vi "DLS Profile.vi"(0 "GEA2 Reference In":refnum<k24>, 1 "Shift To":enum16{"Spin", "Agitate"}(ring), 2 "Input Bit":T3, 5 "GEA Inputs":T4={"Source"=228, "Destination"=192} {"Destination" format="%.0x"; "Source" format="%.0x"}, 7 "Standalone?":bool, 11 "Error In":errorcluster, 12 "Action":enum16{"Lock", "Unlock"}(ring), 13 "Co-efficient Data":T2) -> (4 "GEA2 Reference Out":refnum<k24>, 6 "Calc_Dry Load Size":dbl, 8 "Expected_Dry Load Size":dbl, 10 "Report Text":string, 14 "Pass/Fail":bool, 15 "Error Out":errorcluster)   [LabVIEW 2016, in "TLMB.lvlib"]
uses:
  Projects/TLMB.lvlib
  Q:/Common/DLLs/GEA3/GeaCommunication.dll
  Common/DLLs/GEA3/GeaCommunication.dll
  Common/LabVIEW GEA2 Toolkit/LabVIEW_GEA2_Toolkit.lvlibp/type defs/Source_Destination.ctl
  Control/DLS ERD Data.ctl
  TLMB Common/type defs/Drive Cycle Engine Request State.ctl
  Common/LabVIEW GEA2 Toolkit/LabVIEW_GEA2_Toolkit.lvlibp/type defs/ERD Read Data In.ctl
  Common/LabVIEW GEA2 Toolkit/LabVIEW_GEA2_Toolkit.lvlibp/type defs/Data Type.ctl
  Common/LabVIEW GEA2 Toolkit/LabVIEW_GEA2_Toolkit.lvlibp
panel:
  out "R1_DLS ERD Data":T1
  out "R1_Result Q5 Tranformation":dbl
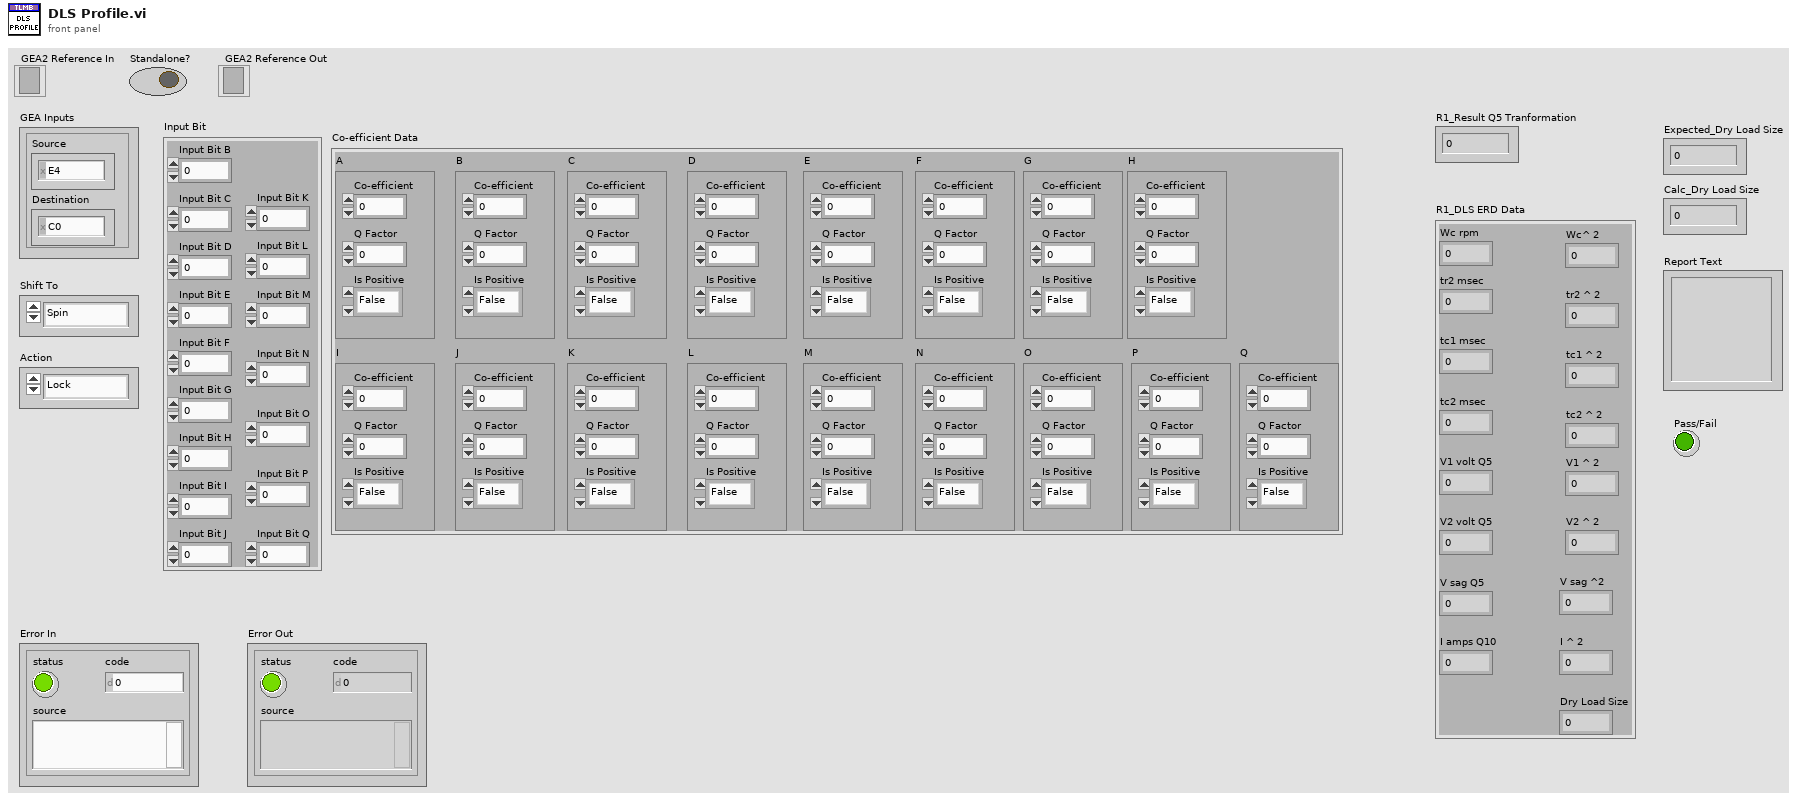
[diagram p1: front panel]
types:
  T1 = typedef "TLMB.lvlib/DLS ERD Data.ctl" = cluster{"Wc rpm":dbl, "tr2 msec":dbl, "tc1 msec":dbl, "tc2 msec":dbl, "V1 volt Q5":dbl, "V2 volt Q5":dbl, "I amps Q10":dbl, "Wc^ 2":dbl, "tr2 ^ 2":dbl, "tc1 ^ 2":dbl, "tc2 ^ 2":dbl, "V1 ^ 2":dbl, "V2 ^ 2":dbl, "I ^ 2":dbl, "V sag Q5":dbl, "V sag ^2":dbl, "Dry Load Size":dbl}
  T2 = cluster{"A":cluster{"Co-efficient":dbl, "Q Factor":dbl, "Is Positive":enum16{"False", "True"}}, "B":cluster{"Co-efficient":dbl, "Q Factor":dbl, "Is Positive":enum16{"False", "True"}}, "C":cluster{"Co-efficient":dbl, "Q Factor":dbl, "Is Positive":enum16{"False", "True"}}, "D":cluster{"Co-efficient":dbl, "Q Factor":dbl, "Is Positive":enum16{"False", "True"}}, "E":cluster{"Co-efficient":dbl, "Q Factor":dbl, "Is Positive":enum16{"False", "True"}}, "F":cluster{"Co-efficient":dbl, "Q Factor":dbl, "Is Positive":enum16{"False", "True"}}, "G":cluster{"Co-efficient":dbl, "Q Factor":dbl, "Is Positive":enum16{"False", "True"}}, "H":cluster{"Co-efficient":dbl, "Q Factor":dbl, "Is Positive":enum16{"False", "True"}}, "I":cluster{"Co-efficient":dbl, "Q Factor":dbl, "Is Positive":enum16{"False", "True"}}, "J":cluster{"Co-efficient":dbl, "Q Factor":dbl, "Is Positive":enum16{"False", "True"}}, "K":cluster{"Co-efficient":dbl, "Q Factor":dbl, "Is Positive":enum16{"False", "True"}}, "L":cluster{"Co-efficient":dbl, "Q Factor":dbl, "Is Positive":enum16{"False", "True"}}, "M":cluster{"Co-efficient":dbl, "Q Factor":dbl, "Is Positive":enum16{"False", "True"}}, "N":cluster{"Co-efficient":dbl, "Q Factor":dbl, "Is Positive":enum16{"False", "True"}}, "O":cluster{"Co-efficient":dbl, "Q Factor":dbl, "Is Positive":enum16{"False", "True"}}, "P":cluster{"Co-efficient":dbl, "Q Factor":dbl, "Is Positive":enum16{"False", "True"}}, "Q":cluster{"Co-efficient":dbl, "Q Factor":dbl, "Is Positive":enum16{"False", "True"}}}
  T3 = cluster{"Input Bit B":dbl, "Input Bit C":dbl, "Input Bit D":dbl, "Input Bit E":dbl, "Input Bit F":dbl, "Input Bit G":dbl, "Input Bit H":dbl, "Input Bit I":dbl, "Input Bit J":dbl, "Input Bit K":dbl, "Input Bit L":dbl, "Input Bit M":dbl, "Input Bit N":dbl, "Input Bit O":dbl, "Input Bit P":dbl, "Input Bit Q":dbl}
  T4 = typedef "LabVIEW_GEA2_Toolkit.lvlibp/Source_Destination.ctl" = cluster{"Source":u8, "Destination":u8}
  T5 = enum16{"EQ (==)", "NE (!=)", "GT (>)", "LT (<)", "GE (>=)", "LE (<=)", "GTLT(> <)", "GELE (>= <=)", "GELT (>= <)", "GTLE (> <=)", "LTGT (< >)", "LEGE (<= >=)", "LEGT (<= >)", "LTGE (< >=)", "No Comparison"}
  T6 = typedef "LabVIEW_GEA2_Toolkit.lvlibp/ERD Read Data In.ctl" = cluster{"ERD Number":u16, "Data Type":T7}
  T7 = typedef "LabVIEW_GEA2_Toolkit.lvlibp/Data Type.ctl" = enum16{"string", "boolean", "uint8_t", "uint16_t", "uint32_t", "uint64_t", "int8_t", "int16_t", "int32_t", "int64_t"}
  T8 = typedef "TLMB.lvlib/Drive Cycle Engine Request State.ctl" = enum16{"Start", "Stop", "Pause", "Resume", "Select"}
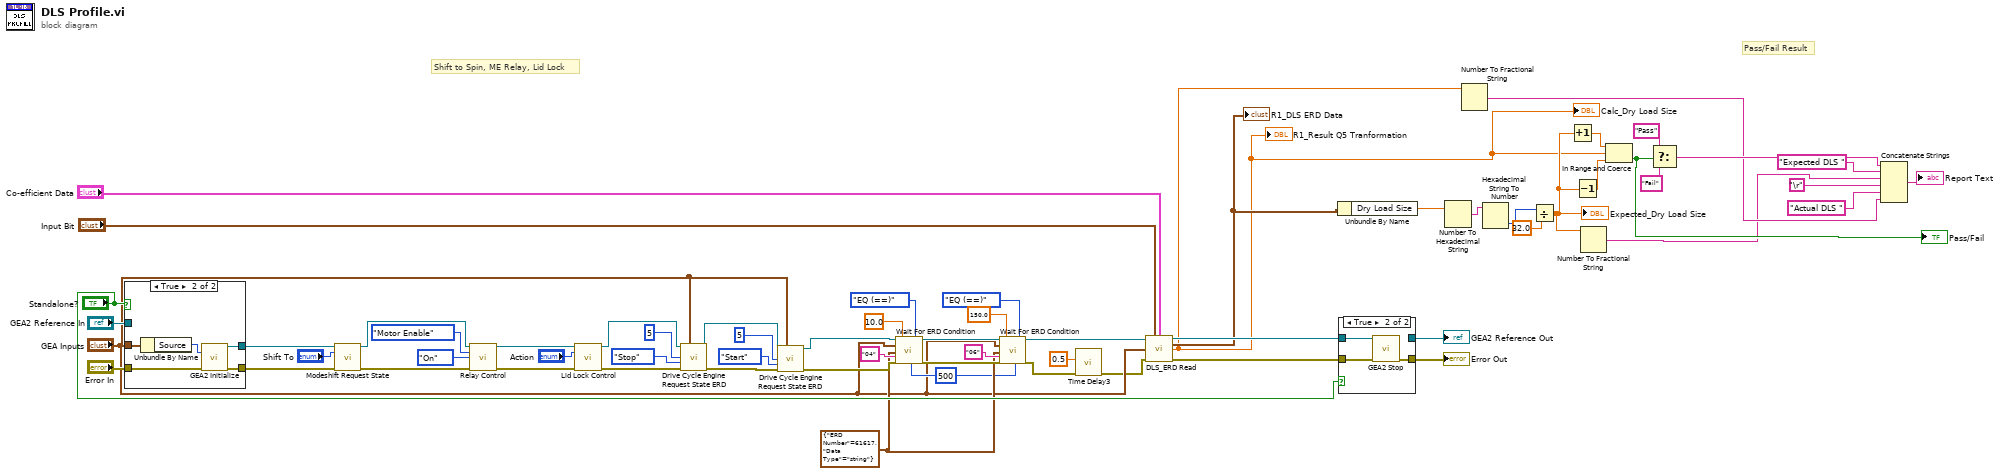
[diagram p0: block diagram]
diagram:
  w29 = u32 500 ("Loop Rate (ms)")
  w32 = T6 {"ERD Number"=61617, "Data Type"=enum."string"} ("ERD Read Data")
  # "Shift to Spin, ME Relay, Lid Lock"
  # "Pass/Fail Result"
  n1 = case shown="True" "Standalone?" {
    tunnel: "GEA2 Reference In" -> [w65 _]
    tunnel: [w65 w70] -> w49
    tunnel: "Error In" -> [w64 w69]
    tunnel: [w64 w68] -> w47
    tunnel: "GEA Inputs" -> [_ w67]
    frame False {
    }
    frame True {
      n2 = Unbundle By Name(w67) -> ("Source"=w66:u8)
      n3 = call "GEA2 Initialize.vi"("Source Address"=w66, "error in"=w69) -> ("GEA2 Reference Out"=w70:refnum<k24>, "error out"=w68:errorcluster)  [unwired: 11 in, 1 out]
    }
  }
  n4 = call "Modeshift Request State.vi"("GEA2 Reference In"=w49, "Shift To"="Shift To", "Error In"=w47) -> ("GEA2 Reference Out"=w48:refnum<k24>, "Error Out"=w46:errorcluster)  [unwired: 9 in, 2 out]
  n5 = call "Relay Control.vi"("GEA2 Reference In"=w48, "Relay"=enum16{"Motor Enable", "Valve", "Both"}."Motor Enable", "State"=enum16{"On", "Off"}."On", "Error In"=w46) -> ("GEA2 Reference Out"=w56:refnum<k24>, "Error Out"=w54:errorcluster)  [unwired: 8 in, 2 out]
  n6 = call "Lid Lock Control.vi"("GEA2 Reference In"=w56, "Action"="Action", "Error In"=w54) -> ("GEA2 Reference Out"=w55:refnum<k24>, "Error Out"=w53:errorcluster)  [unwired: 9 in, 2 out]
  n7 = call "Drive Cycle Engine Request State ERD.vi"("GEA2 Reference In"=w55, "GEA Inputs"="GEA Inputs", "Cycle ID"=u8 5, "Drive Cycle Engine Request State"=Drive_Cycle_Engine_Request_State."Stop", "Error In"=w53) -> ("GEA2 Reference Out"=w44:refnum<k24>, "Error Out"=w43:errorcluster)  [unwired: 9 in]
  n8 = call "Drive Cycle Engine Request State ERD.vi"("GEA2 Reference In"=w44, "GEA Inputs"="GEA Inputs", "Cycle ID"=u8 5, "Drive Cycle Engine Request State"=Drive_Cycle_Engine_Request_State."Start", "Error In"=w43) -> ("GEA2 Reference Out"=w39:refnum<k24>, "Error Out"=w40:errorcluster)  [unwired: 9 in]
  n9 = call "Wait For ERD Condition.vi"("GEA2 Reference In"=w39, "GEA Inputs"="GEA Inputs", "ERD Read Data"=w32, "Expected Low"="04", "Error In"=w40, "Timeout (s)"=10.0, "Loop Rate (ms)"=w29, "Comparison"=T5."EQ (==)") -> ("GEA2 Reference Out"=w35:refnum<k24>, "Error Out"=w34:errorcluster)  [unwired: 7 in, 3 out]
  n10 = call "Wait For ERD Condition.vi"("GEA2 Reference In"=w35, "GEA Inputs"="GEA Inputs", "ERD Read Data"=w32, "Expected Low"="06", "Error In"=w34, "Timeout (s)"=150.0, "Loop Rate (ms)"=w29, "Comparison"=T5."EQ (==)") -> ("GEA2 Reference Out"=w28:refnum<k24>, "Error Out"=w3:errorcluster)  [unwired: 7 in, 3 out]
  n11 = call "Time Delay3"("error in (no error)"=w3, "Delay Time (s)"=0.5) -> ("error out"=w2:errorcluster)  [unwired: 9 in]
  n12 = call "DLS_ERD Read.vi"("GEA2 Reference In"=w28, "Input Bit"="Input Bit", "Co-efficient Data"="Co-efficient Data", "GEA Inputs"="GEA Inputs", "Error In"=w2) -> ("GEA2 Reference Out"=w24:refnum<k24>, "DLS ERD Data"=w22:T1, "Result Q5 Tranformation"=w1:dbl, "Error Out"=w23:errorcluster)  [unwired: 7 in]
  "R1_DLS ERD Data" <- w22
  "R1_Result Q5 Tranformation" <- w1
  "Calc_Dry Load Size" <- w1
  n13 = Unbundle By Name(w22) -> ("Dry Load Size"=w19:dbl)
  n14 = case shown="True" "Standalone?" {
    tunnel: [w71 w75] -> w61
    tunnel: w23 -> [w71 w74]
    tunnel: w24 -> [w72 w73]
    tunnel: [w72 _] -> w58
    frame False {
    }
    frame True {
      n15 = call "GEA2 Stop.vi"("GEA2 Reference In"=w73, "Error In"=w74) -> ("Error Out"=w75:errorcluster)  [unwired: 13 in]
    }
  }
  "GEA2 Reference Out" <- w58
  "Error Out" <- w61
  n16 = Number To Hexadecimal String(2:w19) -> (0:w12:string)  [unwired: 1 in]
  n17 = Number To Fractional String(number=w1) -> (F-format string=w7:string)  [unwired: 3 in]
  n18 = Hexadecimal String To Number(string=w12) -> (number=w21:u32)  [unwired: 2 in, 1 out]
  n19 = Divide(x=w21, y=32.0) -> (x/y=w6:dbl)
  "Expected_Dry Load Size" <- w6
  n20 = Increment(x=w6) -> (x+1=w17:dbl)
  n21 = Decrement(x=w6) -> (x-1=w18:dbl)
  n22 = Number To Fractional String(number=w6) -> (F-format string=w5:string)  [unwired: 3 in]
  n23 = In Range and Coerce(upper limit=w17, x=w1, lower limit=w18) -> (In Range?=w16:bool)  [unwired: 1 out]
  "Pass/Fail" <- w16
  n24 = Select(t="Pass", s=w16, f="Fail") -> (s? t:f=w8:string)
  n25 = Concatenate Strings(w8, "Expected DLS " ("string"), w5, "\r", "Actual DLS " ("string"), w7) -> (→"Report Text":string)
